vi "Port and File Config.vi"() -> (0 "path out":path, 3 "port in":refnum<visa-resource-name>)   [LabVIEW 2014]
panel:
  in  "File Path":path
  in  "Port":refnum<visa-resource-name>="COM3"
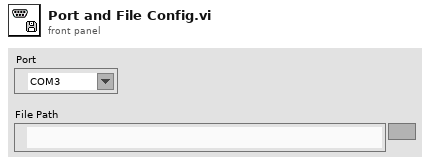
[diagram p1: front panel]
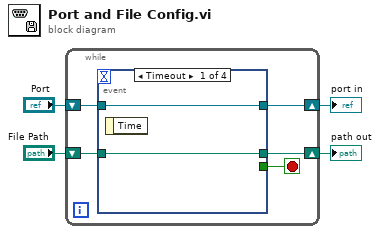
[diagram p0: block diagram]
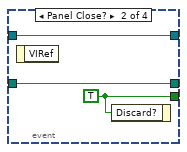
[diagram p2: hidden frame]
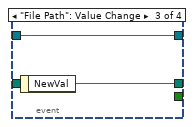
[diagram p3: hidden frame]
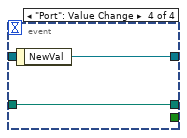
[diagram p4: hidden frame]
diagram:
  n1 = while {
    shift-right: [w6] -> w3
    shift-left: "Port" -> [w9]
    shift-right: [w7] -> w4
    shift-left: "File Path" -> [w8]
    stop <- w5 stop-if-true
    n2 = event shown="[0] Timeout" {
      selector: _ -> [_ _ _ _]
      dyn-events: _ -> [_ _ _ _]
      timeout: _ -> [_ _ _ _]
      tunnel: w9 -> [w11 w14 w16 _]
      tunnel: [w11 w14 w16 w18] -> w6
      tunnel: [w10 w13 w15 w17] -> w7
      tunnel: w8 -> [w10 w13 _ w17]
      tunnel: [_ w12 _ _] -> w5
      event Timeout {
        n3 = event-data() -> ()  [unwired: 1 in, 1 out]
      }
      event Panel Close? {
        w12 = TRUE ("Discard?")
        n4 = event-data() -> ()  [unwired: 1 in, 1 out]
        n5 = event-data("Discard?"=w12) -> ()  [unwired: 1 in, 1 out]
      }
      event "File Path": Value Change {
        n6 = event-data() -> ("NewVal"=w15:path)  [unwired: 1 in]
      }
      event "Port": Value Change {
        n7 = event-data() -> ("NewVal"=w18:refnum<visa-resource-name>)  [unwired: 1 in]
      }
    }
  }
  "path out" <- w4
  "port in" <- w3
